vi "SetLibraryIcon.vi"(8 "error in (no error)":errorcluster, 9 "ApplyIconToVIs (T)":bool=TRUE, 10 "Icon":refnum<class "Icon.lvclass">, 11 "Library":refnum<vi>) -> (0 "error out":errorcluster, 3 "Library out":refnum<vi>)   [LabVIEW 2014, in "ClassIconTools.lvlib"]
uses:
  ClassIconTools.lvlib
  <vilib>/LabVIEW Icon API/lv_icon/Classes/Icon/Icon.lvclass
  <vilib>/LabVIEW Icon API/LabVIEW Icon API.lvlib
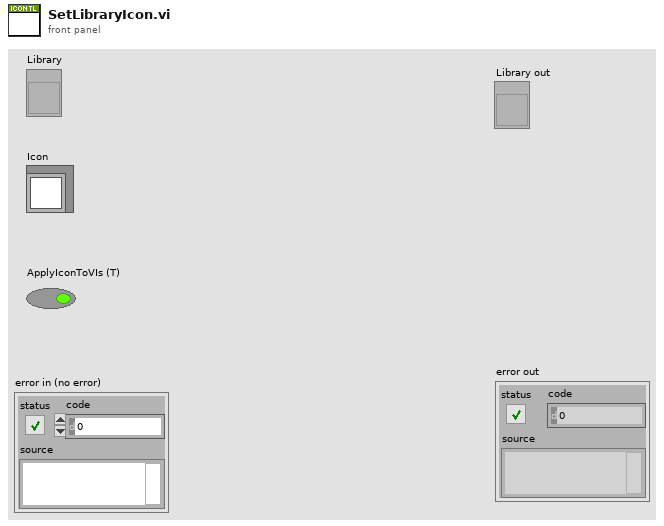
[diagram p1: front panel]
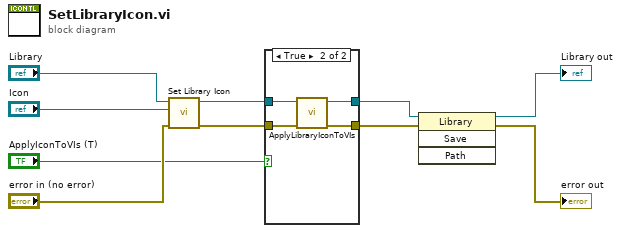
[diagram p0: block diagram]
diagram:
  n1 = call <vilib>:"Set Library Icon.vi"("error in (no error)"="error in (no error)", "Icon"="Icon", "Library Refnum in"="Library") -> ("error out"=w10:errorcluster, "Library Refnum out"=w9:refnum<vi>)  [unwired: 7 in]
  n2 = case shown="True" "ApplyIconToVIs (T)" {
    tunnel: w10 -> [w12 w16]
    tunnel: w9 -> [w11 w15]
    tunnel: [w11 w14] -> w8
    tunnel: [w12 w13] -> w7
    frame False {
    }
    frame True {
      n3 = call "ApplyLibraryIconToVIs.vi"("error in (no error)"=w16, "Library Refnum"=w15) -> ("error out"=w13:errorcluster, "Library Refnum out"=w14:refnum<vi>)  [unwired: 8 in]
    }
  }
  n4 = invoke class="Library" method="Save"(reference=w8, error in=w7) -> (reference out=→"Library out":refnum<vi>, error out=→"error out":errorcluster)  [unwired: 2 in, 2 out]
